vi "IR_error tune while laser on.vi"() -> ()   [LabVIEW 2016]
panel:
  in  "Stop":bool
  # "Error: laser (Q-switch) is on)"
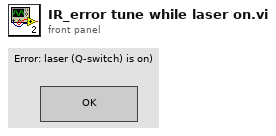
[diagram p1: front panel]
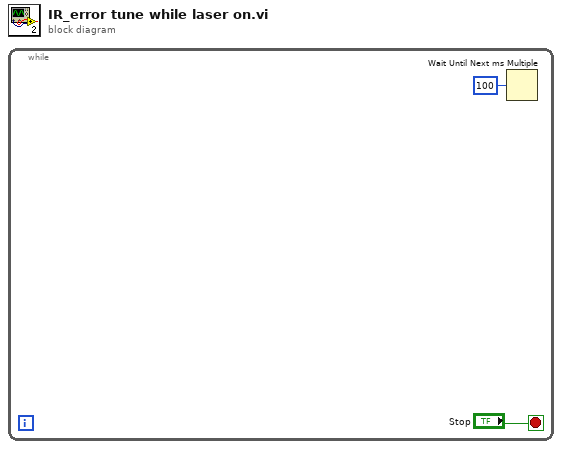
[diagram p0: block diagram]
diagram:
  n1 = while {
    stop <- "Stop" stop-if-true
    n2 = Wait Until Next ms Multiple(millisecond multiple=u32 100) -> ()  [unwired: 1 out]
  }
